vi "KIM_InitDone.vi"(8 "error in (no error)":errorcluster, 10 "KIM Positions":T1, 11 "TranslationStageUI.lvclass":refnum<class "TranslationStageUI.lvclass">) -> (0 "error out":errorcluster, 3 "TranslationStageUI.lvclass":refnum<class "TranslationStageUI.lvclass">)   [LabVIEW 2023, in "TranslationStage_UI.lvlib" / "TranslationStageUI.lvclass"]
uses:
  TranslationStageUI.lvclass
  BPC_Voltages.ctl
  TranslationStageUI.lvclass/TranslationStageUI.ctl
  typedefs/typedefs.lvlib
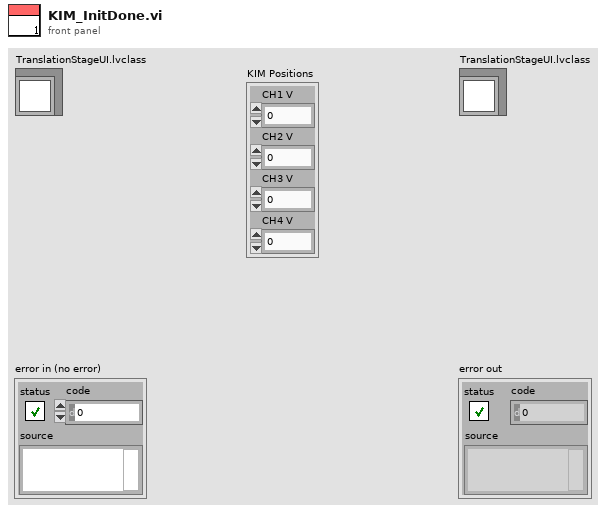
[diagram p1: front panel]
types:
  T1 = typedef "typedefs.lvlib/BPC_Voltages.ctl" = cluster{"CH1 V":i32, "CH2 V":i32, "CH3 V":i32, "CH4 V":i32}
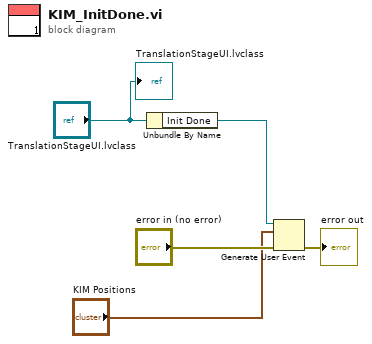
[diagram p0: block diagram]
diagram:
  n1 = Unbundle By Name("TranslationStageUI.lvclass") -> ("Init Done"=w5:refnum<user-event>)
  n2 = Generate User Event(user event=w5, event data cluster="KIM Positions", error in="error in (no error)") -> (error out=→"error out":errorcluster)  [unwired: 1 in, 1 out]
  "TranslationStageUI.lvclass" <- "TranslationStageUI.lvclass"
